vi "K2400_setCURR.vi"(2 "error in (no error)":errorcluster, 3 "Current [A]":dbl, 4 "GPIB address":refnum<visa-resource-name>) -> (0 "error out":errorcluster, 1 "VISA resource name out":refnum<visa-resource-name>)   [LabVIEW 2011]
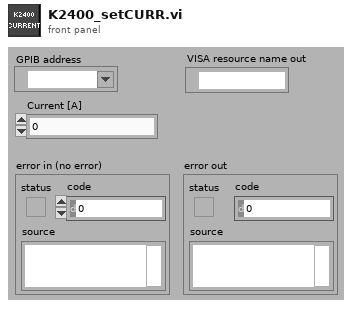
[diagram p1: front panel]
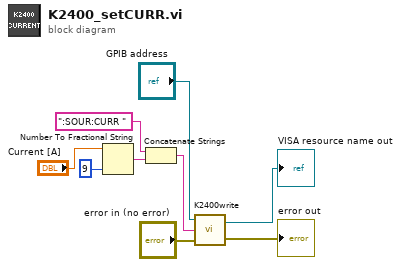
[diagram p0: block diagram]
diagram:
  n1 = Number To Fractional String(number="Current [A]", precision (6)=9) -> (F-format string=w6:string)  [unwired: 2 in]
  n2 = Concatenate Strings(":SOUR:CURR ", w6) -> (w5:string)
  n3 = call "K2400write.vi"("error in (no error)"="error in (no error)", "Command"=w5, "VISA Resource Name"="GPIB address") -> ("error out"=→"error out":errorcluster, "VISA resource name out"=→"VISA resource name out":refnum<visa-resource-name>)
